vi "Sensoren_buendeln.vi"(0 "rechts seite":dbl, 1 "rechts geradeaus":dbl, 2 "rechts Schräg":dbl, 3 "Links schräg":dbl, 4 "Links Geradeaus":dbl, 5 "Links seite":dbl, 6 "rechts hinten":dbl, 8 "links hinten":dbl) -> (7 "SensorArray":dbl[](array[numeric]))   [LabVIEW 2016]
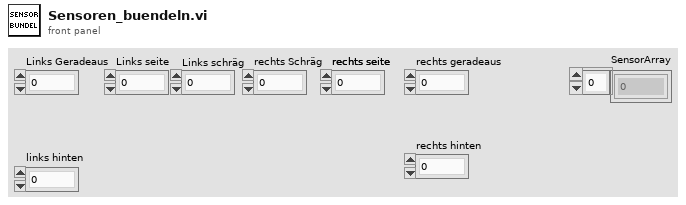
[diagram p1: front panel]
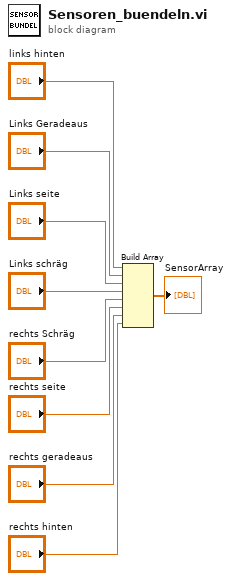
[diagram p0: block diagram]
diagram:
  n1 = Build Array("links hinten", "Links Geradeaus", "Links seite", "Links schräg", "rechts Schräg", "rechts seite", "rechts geradeaus", "rechts hinten") -> (→"SensorArray":dbl[])
